vi "store_mem_current_pos.vi"(8 "error in (no error)":errorcluster, 9 "storage_id":i32, 10 "device ID":i32, 11 "Handle in":i64) -> (0 "error out":errorcluster, 2 "Return (<0 is error)":i32, 3 "Handle out":i64)   [LabVIEW 2016, in "OSB_uMp_library.lvlib"]
doc: "Store uMp's current position"
uses:
  OSB_uMp_library.lvlib
  ump.dll
panel:
  # "By Stuart Box at OxSyBio Ltd, 2017\n\nThis software is provided WITHOUT ANY WARRANTY; without even the implied warranty of MERCHANTABILITY or FITNESS FOR A PARTICULAR PURPOSE.\n\ninfo@oxsybio.com\n\nOxSyBio Ltd, The Walbrook Building, 25 Walbrook, London, EC4N 8AF"
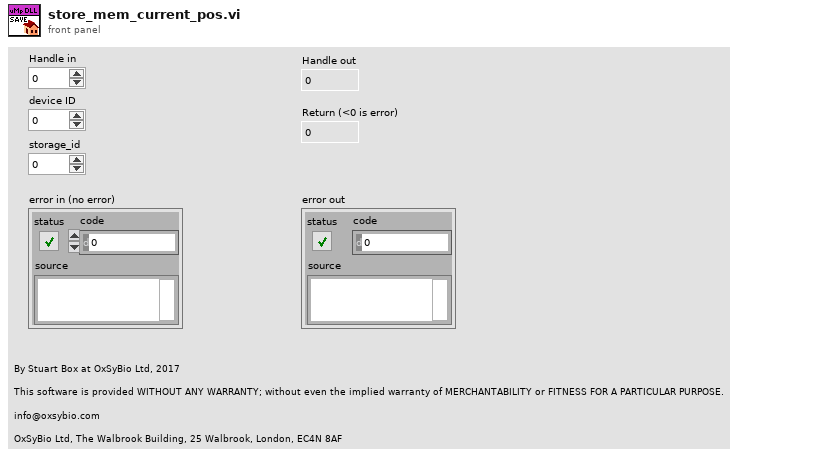
[diagram p1: front panel]
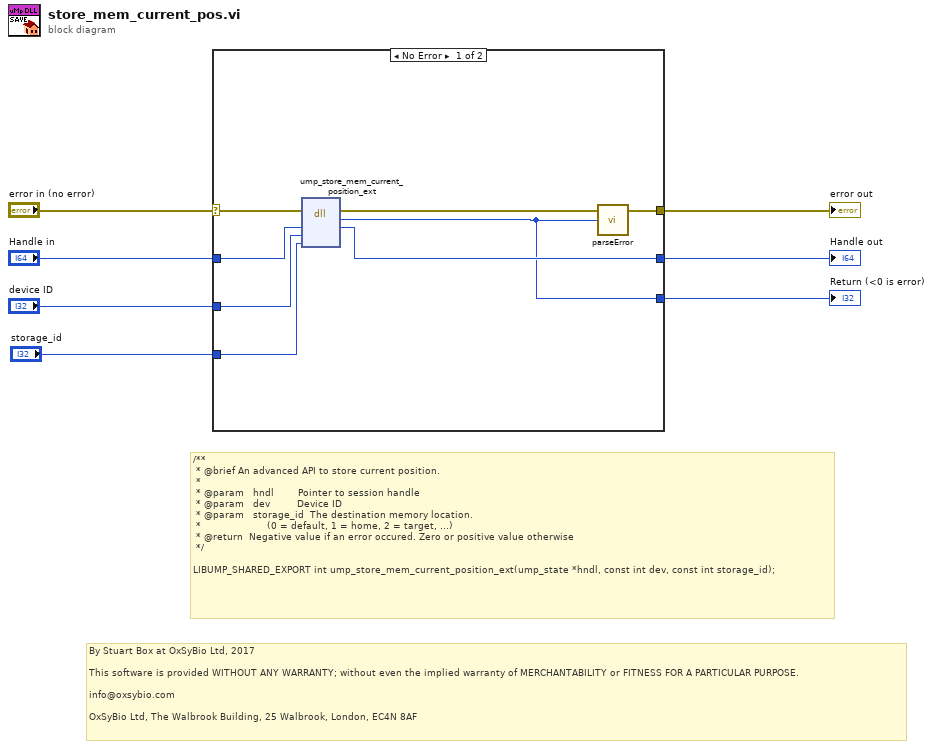
[diagram p0: block diagram]
diagram:
  # "By Stuart Box at OxSyBio Ltd, 2017\n\nThis software is provided WITHOUT ANY WARRANTY; without even the implied warranty of MERCHANTABILITY or FITNESS FOR A PARTICULAR PURPOSE.\n\ninfo@oxsybio.com\n\nOxSyBio Ltd, The Walbrook Building, 25 Walbrook, London, EC4N 8AF"
  # "/**\n * @brief An advanced API to store current position.\n *\n * @param   hndl        Pointer to session handle\n * @param   dev         Device ID\n * @param   storage_id  The destination memory location.\n *                      (0 = default, 1 = home, 2 = target, ...)\n * @return  Negative value if an error occured. Zero or positive value otherwise\n */\n\nLIBUMP_SHARED_EXPORT int ump_store_mem_current_position_ext(ump_state *hndl, const int dev, const int storage_id);"
  n1 = case shown="No Error" "error in (no error)" {
    selector: "error in (no error)" -> [w11 w17]
    tunnel: [w15 w16] -> w7
    tunnel: "storage_id" -> [w14 _]
    tunnel: "device ID" -> [w13 _]
    tunnel: [w9 w17] -> w4
    tunnel: [w8 _] -> w3
    tunnel: "Handle in" -> [w12 w16]
    frame No Error {
      n2 = dll-call lib="C:/Users/Stu/Desktop/OSB LabVIEW uMp/uMp_library/ump.dll" fn="ump_store_mem_current_position_ext"(error in=w11, "handle"=w12, "dev"=w13, "storage_id"=w14) -> (error out=w10:errorcluster, "return"=w8:i32, "handle"=w15:i64)  [unwired: 4 in, 1 out]
      n3 = call "parseError.vi"("Error In"=w10, "ump dll return value (<0 is error)"=w8) -> ("Error Out"=w9:errorcluster)  [unwired: 24 in, 1 out]
    }
    frame Error {
    }
  }
  "Handle out" <- w7
  "error out" <- w4
  "Return (<0 is error)" <- w3
